vi "Validate Range.vi"(8 "error in (no error)":errorcluster, 11 "Magnetic Field in":refnum<class "Magnetic Field.lvclass">) -> (0 "error out":errorcluster, 3 "Magnetic Field out":refnum<class "Magnetic Field.lvclass">)   [LabVIEW 2009, in "Magnetic Field.lvclass"]
doc: "Coerce the range to be within this Scanner's physical limits."
uses:
  Magnetic Field.lvclass
  Scanner/Scanner.lvclass
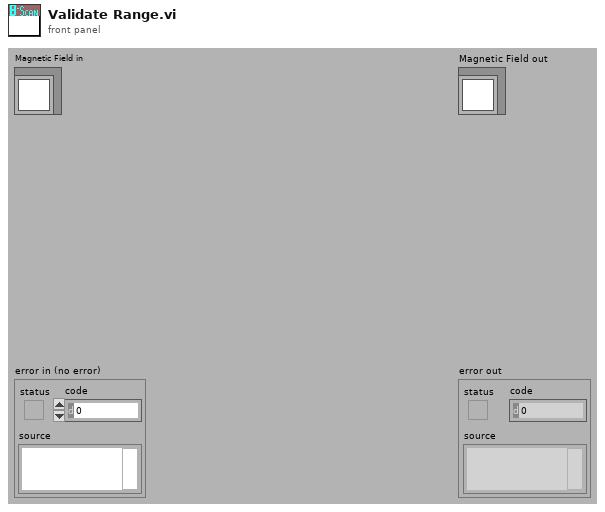
[diagram p1: front panel]
types:
  T1 = typedef "Scanner.lvclass/Range.ctl" = cluster{"xi":dbl, "xf":dbl, "dx":dbl, "Return to...?":bool, "Return to":dbl}
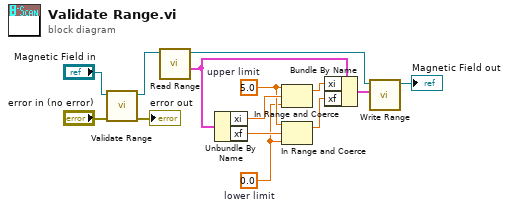
[diagram p0: block diagram]
diagram:
  w7 = 0.0  # lower limit
  w8 = 5.0  # upper limit
  n1 = call-parent "Validate Range.vi"("error in (no error)"="error in (no error)", "Scanner in"="Magnetic Field in") -> ("error out"=→"error out":errorcluster, "Scanner out"=w11:refnum<class "Magnetic Field.lvclass">)  [unwired: 8 in]
  n2 = call-dynamic "Read Range.vi"("Scanner.lvclass in"=w11) -> ("Range"=w5:T1, "Scanner.lvclass out"=w2:refnum<class "Magnetic Field.lvclass">)  [unwired: 5 in, 4 out]
  n3 = Unbundle By Name(w5) -> ("xi"=w10:dbl, "xf"=w9:dbl)
  n4 = In Range and Coerce(upper limit=w8, x=w10, lower limit=w7) -> (coerced(x)=w4:dbl)  [unwired: 1 out]
  n5 = In Range and Coerce(upper limit=w8, x=w9, lower limit=w7) -> (coerced(x)=w3:dbl)  [unwired: 1 out]
  n6 = Bundle By Name(cluster=w5, "xi"=w4, "xf"=w3) -> (w6:T1)
  n7 = call-dynamic "Write Range.vi"("Range"=w6, "Scanner in"=w2) -> ("Scanner out"=→"Magnetic Field out":refnum<class "Magnetic Field.lvclass">)  [unwired: 7 in, 2 out]
